vi "BodeMagnitudePlot.vi"() -> ()   [LabVIEW 2015]
uses:
  <vilib>/imath/engines/lvmath2/RunTimeEngine/Managers/WorkSpace/UID Generator.vi
  <vilib>/imath/engines/lvmath2/RunTimeEngine/RunTimeType/NIMS_RunTimeType_From StrictType (excl LVString).vi
  <instcachedir>/0/NIMS_RunTimeType_From StrictType (excl LVString)_EB1C38A9BC5048DA9ABDA8F781E54D21.lvgen/NIMS_RunTimeType_From StrictType (excl LVString)_EB1C38A9BC5048DA9ABDA8F781E54D21_000.vi
  <vilib>/imath/engines/lvmath2/RunTimeEngine/LocalVariableDefStatement/MC_LocalVariableDefStatement_Display.vi
  <vilib>/imath/engines/lvmath2/RunTimeEngine/Managers/SymbolTable/Clear UID.vi
  <vilib>/imath/engines/lvmath2/RunTimeEngine/NodeEndStatement/NIMS_NodeEndStatement_Output.vi
  <instcachedir>/0/NIMS_NodeEndStatement_Output_53EC0D466D134D7ABD903AC30B43404B.lvgen/NIMS_NodeEndStatement_Output_53EC0D466D134D7ABD903AC30B43404B_005.vi
  <vilib>/imath/engines/lvmath2/RunTimeEngine/ErrorHandling/NIMS_Finalize Error.vi
  <vilib>/Analysis/NI_AALPro.lvlib
  <vilib>/imath/engines/lvmath2/RunTimeEngine/Managers/SymbolTable/NIMS_WorkSpace.lvlib
panel:
  out "XY Graph":cluster{"X":dbl, "Y":dbl}[](graph)
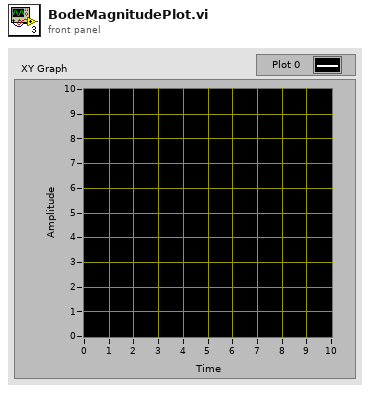
[diagram p1: front panel]
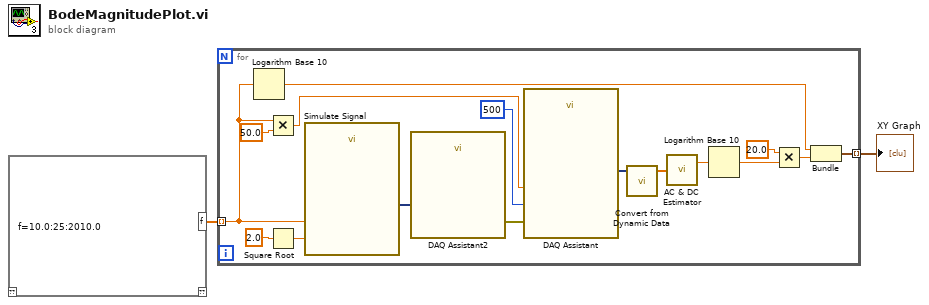
[diagram p0: block diagram]
diagram:
  n1 = mathscript code="f=10.0:25:2010.0"() -> ("f"=w2:dbl[])  [unwired: 1 in, 1 out]
  n2 = for {
    tunnel: w2 -> [w8] mode=indexing
    tunnel: [w5] -> w1 mode=indexing
    n3 = Logarithm Base 10(1:w8) -> (0:w6:dbl)
    n4 = Multiply(x=w8, y=50.0) -> (x*y=w13:dbl)
    n5 = Square Root(x=2.0) -> (sqrt(x)=w11:dbl)
    n6 = call "Simulate Signal"("Frequency"=w8, "Amplitude"=w11) -> ("Sine"=w17:dynamicdata)  [unwired: 12 in, 1 out]
    n7 = call "DAQ Assistant2"("data"=w17) -> ("error out"=w16:errorcluster)  [unwired: 16 in, 2 out]
    n8 = call "DAQ Assistant"("rate"=w13, "number of samples"=500, "error in"=w16) -> ("data"=w12:dynamicdata)  [unwired: 14 in, 2 out]
    n9 = call "Convert from Dynamic Data"("Dynamic Data Type"=w12) -> ("Array"=w4:dbl[])  [unwired: 3 in]
    n10 = call <vilib>:"AC & DC Estimator.vi"("Signal (V)"=w4) -> ("AC estimate (Vrms)"=w3:dbl)  [unwired: 1 out]
    n11 = Logarithm Base 10(1:w3) -> (0:w10:dbl)
    n12 = Multiply(x=20.0, y=w10) -> (x*y=w7:dbl)
    n13 = Bundle(w6, w7) -> (w5:cluster{dbl, dbl})  [unwired: 1 in]
  }
  "XY Graph" <- w1
